vi "run.vi"(8 "error in (no error)":errorcluster, 11 "ErrorController in":refnum<class "ErrorController.lvclass">) -> (0 "error out":errorcluster, 3 "ErrorController out":refnum<class "ErrorController.lvclass">)   [LabVIEW 2010, in "ErrorController.lvclass"]
uses:
  ErrorController.lvclass
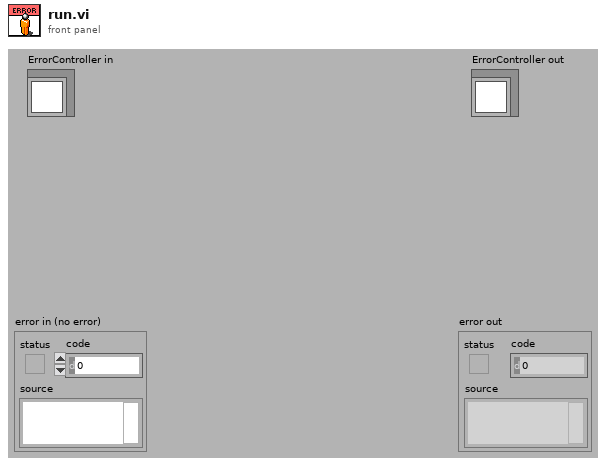
[diagram p1: front panel]
types:
  T1 = typedef "ErrorController.lvclass/error_cluster.ctl" = cluster{"error out":errorcluster, "call chain":string[], "additional message":string, "terminate?":bool, "concatenated string":string}
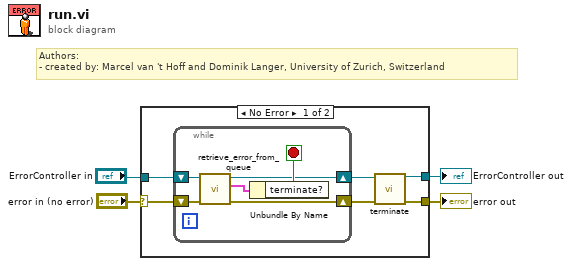
[diagram p0: block diagram]
diagram:
  # "Authors: \n- created by: Marcel van 't Hoff and Dominik Langer, University of Zurich, Switzerland"
  n1 = case shown="No Error" "error in (no error)" {
    selector: "error in (no error)" -> [w6 w17]
    tunnel: [w9 w17] -> w3
    tunnel: [w7 w16] -> w1
    tunnel: "ErrorController in" -> [w5 w16]
    frame No Error {
      n2 = while {
        shift-right: [w12] -> _
        shift-left: w6 -> [w15]
        shift-right: [w10] -> w8
        shift-left: w5 -> [w11]
        stop <- w13 stop-if-true
        n3 = call-dynamic "retrieve_error_from_queue.vi"("error in (no error)"=w15, "ErrorController in"=w11) -> ("error out"=w12:errorcluster, "error information"=w14:T1, "ErrorController out"=w10:refnum<class "ErrorController.lvclass">)  [unwired: 7 in]
        n4 = Unbundle By Name(w14) -> ("terminate?"=w13:bool)
      }
      n5 = call-dynamic "terminate.vi"("error in (no error)"=w6, "ErrorController in"=w8) -> ("error out"=w9:errorcluster, "ErrorController out"=w7:refnum<class "ErrorController.lvclass">)  [unwired: 8 in]
    }
    frame Error {
    }
  }
  "error out" <- w3
  "ErrorController out" <- w1
